vi "Set Splitter Color.vi"(8 "error in (no error)":errorcluster, 10 "Splitter Refnum":refnum<vi>, 11 "OwningVI":refnum<vi>) -> (0 "error out":errorcluster)   [LabVIEW 2017, in "XGrapher.xctl"]
doc: "So here's the deal, the Timeline and regular Graphs are split with a splitter. You can't make splitters invisible, so when the xcontrol starts running, I check the calling VI's background color and set the splitter color to that color (so it looks invisible). \n\nMan, that's fancy."
uses:
  XGrapher.xctl
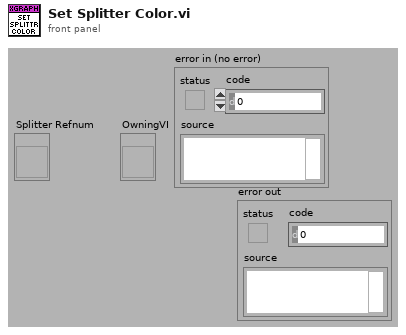
[diagram p1: front panel]
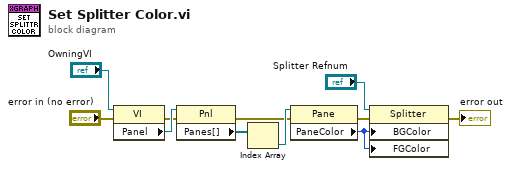
[diagram p0: block diagram]
diagram:
  n1 = property class="VI"(reference="OwningVI", error in="error in (no error)") -> (error out=w4:errorcluster, "Panel"=w8:refnum<vi>)  [unwired: 1 out]
  n2 = property class="Pnl"(reference=w8, error in=w4) -> (error out=w3:errorcluster, "Panes[]"=w9:refnum<vi>[])  [unwired: 1 out]
  n3 = Index Array(array=w9) -> (element=w10:refnum<vi>)  [unwired: 1 in]
  n4 = property class="Pane"(reference=w10, error in=w3) -> (error out=w2:errorcluster, "PaneColor"=w11:u32)  [unwired: 1 out]
  n5 = property on="Property Node" class="Splitter"(reference="Splitter Refnum", error in=w2, "BGColor"=w11, "FGColor"=w11) -> (error out=→"error out":errorcluster)  [unwired: 1 out]
